vi "Current Sensor Callibaration.vi"() -> ()   [LabVIEW 2015]
panel:
  out "Pre Multipication factor":dynamicdata(graph) caption="data"
  out "Waveform Graph":dynamicdata(graph)
  out "RMS 2":dbl
  out "Peak to Peak 2":dbl
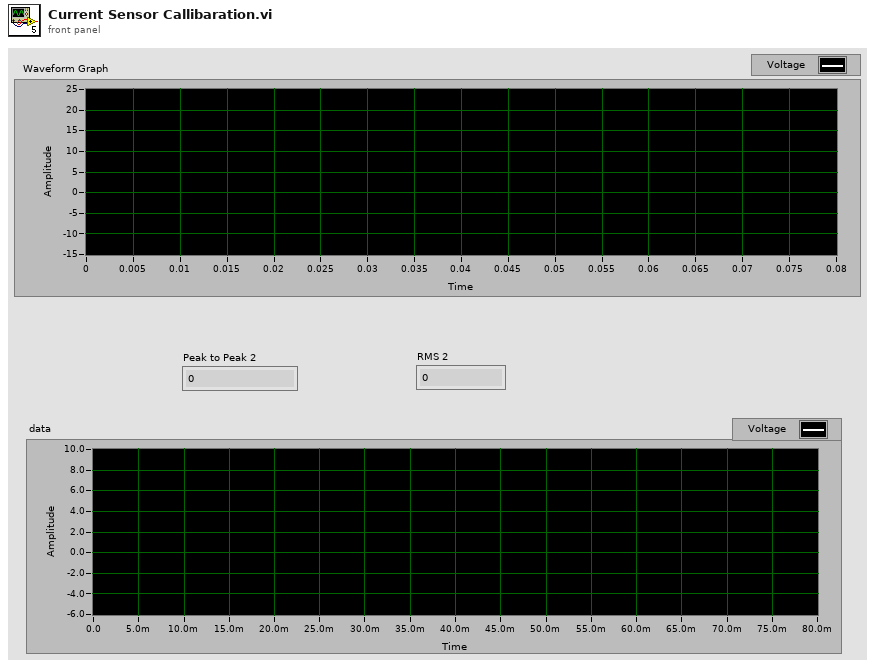
[diagram p1: front panel]
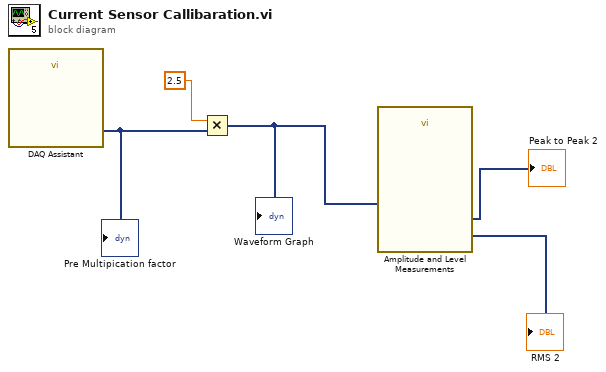
[diagram p0: block diagram]
diagram:
  n1 = call "DAQ Assistant"() -> ("data"=w4:dynamicdata)  [unwired: 17 in, 2 out]
  "Pre Multipication factor" <- w4
  n2 = Multiply(x=2.5, y=w4) -> (x*y=w3:dynamicdata)
  "Waveform Graph" <- w3
  n3 = call "Amplitude and Level Measurements"("Signals"=w3) -> ("RMS"=→"RMS 2":dynamicdata, "Peak to Peak"=→"Peak to Peak 2":dynamicdata)  [unwired: 12 in, 1 out]
